vi "Hong_Correlations.vi"() -> (5 "Plug in titles":string[](array[string]), 7 "Plug in values":string[](array[string]))   [LabVIEW 2010]
uses:
  Globals/Meas_global.vi
  Globals/Plug_in_data_global.vi
panel:
  out "Waveform Graph":dbl[](graph)
  in  "Number of delta T":i32=30
  in  "Inst 2 Index":i32=2
  in  "Inst 1 Index":i32=1
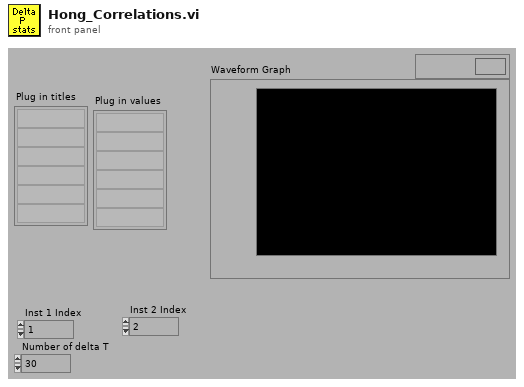
[diagram p1: front panel]
types:
  T1 = typedef "Analysis_info_cluster.ctl" = cluster{"Colour":u32, "Inst type":T2, "Inst name":string, "Symbol":string, "Code name":string, "Extra Info":string, "Inst Array":T3, "Index":i32, "Voltage Index":i32, "Extra Titles":string[], "Extra Values":string[]}
  T2 = typedef "Inst_type.ctl" = enum16{"Propeller anemometer", "Raw voltage", "Pressure Transducer", "Pitot-static tube", "Preston tube", "Hot wire", "Cross wire 1", "Cross wire 2", "Generic Linear", "Generic Polynomial", "Generic BackPoly", "Fast FID", "Thermocouple", "Cold wire", "Pulsed Wire", "LDA Vel", "LDA Tran time", "LDA Arr time"}
  T3 = typedef "Instrument_Array.ctl" = enum16{"PWA", "LDA", "Analogue"}
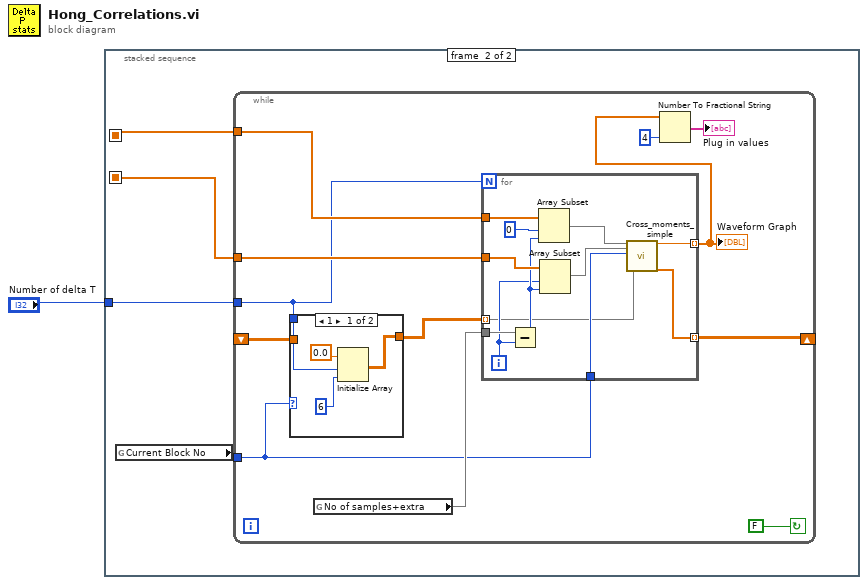
[diagram p0: block diagram]
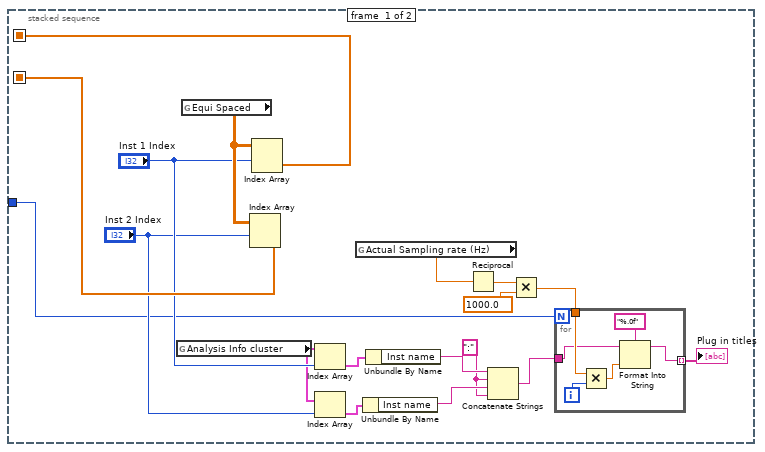
[diagram p2: hidden frame]
diagram:
  n1 = stacked-sequence {
    seq-local: [w17 _] -> [_ w29]
    seq-local: [w18 _] -> [_ w27]
    tunnel: "Number of delta T" -> [w2 w26]
    frame #0 {
      w6 = ":" ("Substring")
      n2 = global read "Meas_global.vi" "Analysis Info cluster"() -> (w14:T1[])
      n3 = global read "Plug_in_data_global.vi" "Equi Spaced"() -> (w19:dbl[][])
      n4 = Index Array(array=w19, index (row)="Inst 2 Index") -> (element=w17:dbl[])  [unwired: 1 in]
      n5 = Index Array(array=w19, index (row)="Inst 1 Index") -> (element=w18:dbl[])  [unwired: 1 in]
      n6 = Index Array(array=w14, index="Inst 1 Index") -> (element=w13:T1)
      n7 = Index Array(array=w14, index="Inst 2 Index") -> (element=w12:T1)
      n8 = global read "Meas_global.vi" "Actual Sampling rate (Hz)"() -> (w11:dbl)
      n9 = Unbundle By Name(w12) -> ("Inst name"=w7:string)
      n10 = Unbundle By Name(w13) -> ("Inst name"=w8:string)
      n11 = Reciprocal(x=w11) -> (1/x=w10:dbl)
      n12 = Concatenate Strings(w8, w6, w7, w6) -> (w5:string)
      n13 = Multiply(x=w10, y=1000.0) -> (x*y=w4:dbl)
      n14 = for {
        N: w2 -> [_]
        tunnel: w5 -> [w23]
        tunnel: w4 -> [w24]
        tunnel: [w20] -> w3 mode=indexing
        i -> [w25]
        n15 = Multiply(x=w24, y=w25) -> (x*y=w22:dbl)
        n16 = Format Into String(format string="%.0f" ("Format String"), initial string=w23, w22) -> (resulting string=w20:string)  [unwired: 1 in, 1 out]
      }
      "Plug in titles" <- w3
    }
    frame #1 {
      n17 = global read "Meas_global.vi" "Current Block No"() -> (w28:i32)
      n18 = while {
        tunnel: w27 -> [w38]
        tunnel: w28 -> [w34]
        tunnel: w26 -> [w35]
        shift-left: _ -> [w37]
        shift-right: [w39] -> _
        tunnel: w29 -> [w40]
        stop <- FALSE continue-if-true
        n19 = case shown="1" w34 {
          tunnel: w35 -> [w44 _]
          tunnel: [w42 w46] -> w36
          tunnel: w37 -> [_ w46]
          frame 1 {
            n20 = Initialize Array(0.0, w44, 6 ("Dimension Size")) -> (w42:dbl[][])
          }
          frame 2, Default {
          }
        }
        n21 = global read "Meas_global.vi" "No of samples+extra"() -> (w41)
        n22 = for {
          N: w35 -> [_]
          tunnel: w38 -> [w58]
          tunnel: w41 -> [w57]
          tunnel: w40 -> [w56]
          tunnel: w34 -> [w50]
          tunnel: [w49] -> w39 mode=indexing
          tunnel: w36 -> [w48] mode=indexing
          tunnel: [w47] -> w32 mode=indexing
          i -> [w53]
          n23 = Subtract(x=w57, y=w53) -> (x-y=w55:i32)
          n24 = Array Subset(array=w58, index=0 ("Array Index"), length=w55) -> (w52:dbl[])
          n25 = Array Subset(array=w56, index=w53, length=w55) -> (w51:dbl[])
          n26 = call "Cross_moments_simple.vi"("U"=w52, "W"=w51, "Block No"=w50, "Shift in"=w48) -> ("Correlation"=w47:dbl, "Shift out"=w49:dbl[])  [unwired: 14 in]
        }
        "Waveform Graph" <- w32
        n27 = Number To Fractional String(number=w32, precision (6)=i16 4) -> (F-format string=→"Plug in values":string[])  [unwired: 2 in]
      }
    }
  }
